vi "Digital Pattern Gen 1.3 FPGA Settings Write Node.vi"(8 "error in (no error)":errorcluster, 10 "settings":T2, 11 "Refnum in":T1) -> (0 "error out":errorcluster, 3 "Refnum out":T1)   [LabVIEW 2015, in "Engine Simulation Toolkit Engine.lvlib"]
uses:
  Engine Simulation Toolkit Engine.lvlib
  Digital Pattern Gen 1.3 Settings Ref.ctl
  <vilib>/rvi/errors/niLvFpgaAdjustHostInterfaceError.vi
  <vilib>/Utility/error.llb/Error Cluster From Error Code.vi
  <vilib>/rvi/interface/nirviReadWriteControl/nirviReadWriteControl.xnode
  NiFpgaLv.dll
  <vilib>/rvi/interface/Simulation/niFpgaSimulationCallBeginRW.vi
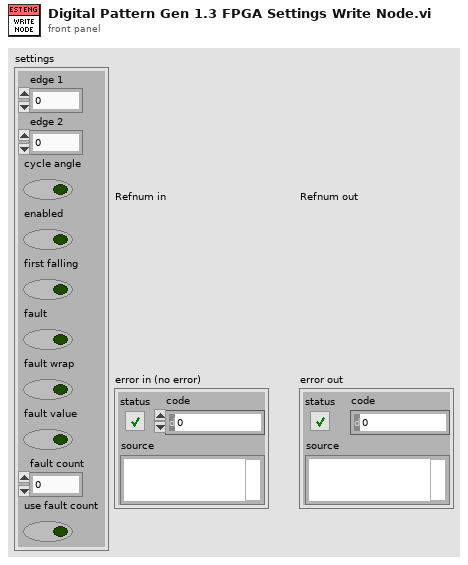
[diagram p1: front panel]
types:
  T1 = typedef "Engine Simulation Toolkit Engine.lvlib/Digital Pattern Gen 1.3 Settings Ref.ctl" = refnum<k20>
  T2 = cluster{"edge 1":u16, "edge 2":u16, "cycle angle":bool, "enabled":bool, "first falling":bool, "fault":bool, "fault wrap":bool, "fault value":bool, "fault count":fxp<+,4,4>, "use fault count":bool}
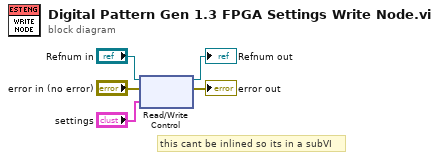
[diagram p0: block diagram]
diagram:
  # "this cant be inlined so its in a subVI"
  n1 = xnode "Read/Write Control"("FPGA VI Reference In"="Refnum in", "error in"="error in (no error)", "Value"="settings") -> ("FPGA VI Reference Out"=→"Refnum out":T1, "error out"=→"error out":errorcluster)
